vi "_PC_Pub_ExpCondiValue_TMP.vi"(2 "error in (no error)":errorcluster, 3 "expCondiVariant":variant) -> (0 "error out":errorcluster, 1 "TMP":T1)   [LabVIEW 2018]
uses:
  <vilib>/Utility/error.llb/Error Cluster From Error Code.vi
  <vilib>/ErrorRing/Error Ring.xnode
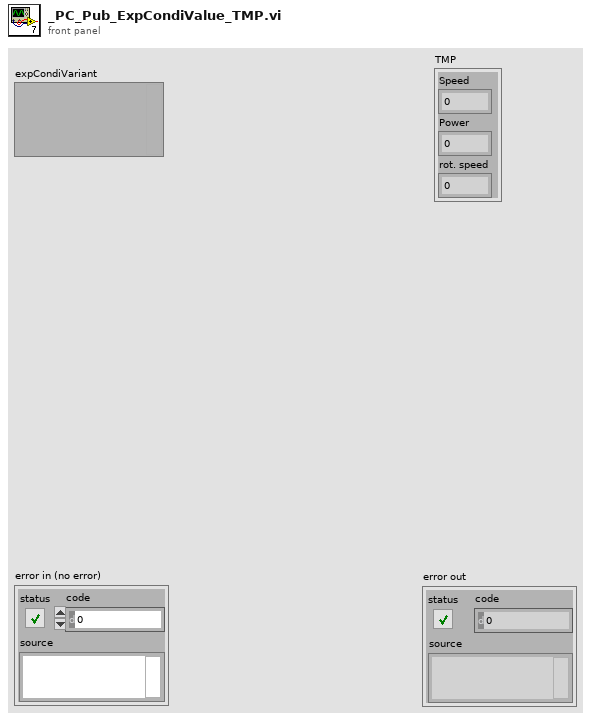
[diagram p1: front panel]
types:
  T1 = cluster{"Speed":dbl, "Power":dbl, "rot. speed":dbl}
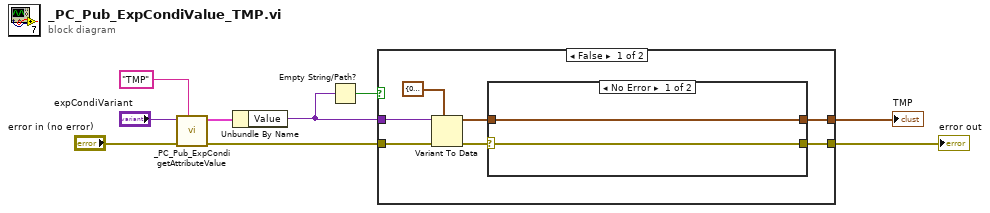
[diagram p0: block diagram]
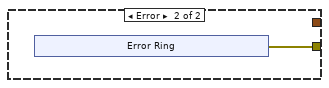
[diagram p2: hidden frame]
diagram:
  n1 = call "_PC_Pub_ExpCondi getAttributeValue.vi"("attrName"="TMP", "error in (no error)"="error in (no error)", "expCondiVariant"="expCondiVariant") -> ("error out"=w7:errorcluster, "attrValue"=w9:cluster{"Label":string, "Value":variant})  [unwired: 7 in]
  n2 = Unbundle By Name(w9) -> ("Value"=w2:variant)
  n3 = Empty String/Path?(string/path=w2) -> (empty?=w1:bool)
  n4 = case shown="False" w1 {
    tunnel: w7 -> [w16 w24]
    tunnel: [w12 _] -> w5
    tunnel: [w11 w24] -> w4
    tunnel: w2 -> [w10 _]
    frame False {
      n5 = Variant To Data(error in=w16, type=T1 {"Speed"=0.0, "Power"=0.0, "rot. speed"=0.0} ("TMP"), Variant=w10) -> (data=w14:T1, error out=w15:errorcluster)
      n6 = case shown="No Error" w15 {
        selector: w15 -> [w17 _]
        tunnel: w14 -> [w18 _]
        tunnel: [w18 _] -> w12
        tunnel: [w17 w19] -> w11
        frame No Error {
        }
        frame Error {
          n7 = xnode "Error Ring"() -> ("error out"=w19:errorcluster)
        }
      }
    }
    frame True {
    }
  }
  "error out" <- w4
  "TMP" <- w5
